vi "NT Globals.vi"() -> ()   [LabVIEW 2025]
panel:
  in  "NT Topics":string[](array[string])
  in  "Update Time":i32=100
  in  "Write Operations":i32
  in  "Read Operations":i32
  in  "Bytes Transmitted":i32
  in  "Updates":i32
  in  "Start Time":timestamp
  in  "Variable Count":i32
  in  "Name":string
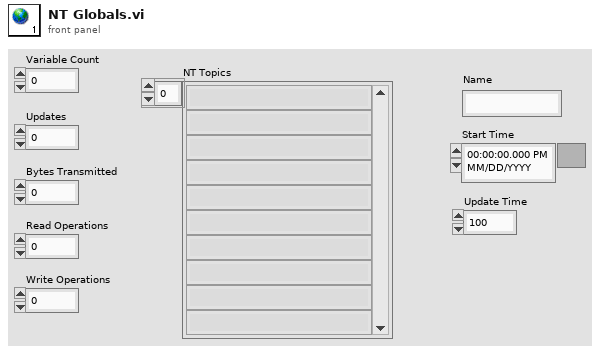
[diagram p1: front panel]
diagram:
